vi "StringHeaderToCluster_v2(SubVI).vi"(8 "error in":errorcluster, 10 "UNDT_Cluster in":T1 {"Gain Coeff" format="%#_6e"; "Reserve 1" format="%02x"; "Mux TX" format="%02x"; "Mux RX" format="%02x"; "ScanDelay" format="%02x"; "PacketCounter" format="%08x"; "SamplingInterval" format="%#_6e"; "Lose Packet" format="%08x"; "EncodersParam2" format="%016x"; "EncodersParam1" format="%016x"; "CRC 8" format="%02x"; "N chanel" format="%02x"; "N tick" format="%02x"; "Ncycle" format="%04x"; "FrameFormatVersion" format="%02x"; "MagicWord" format="%.0x"}, 11 "string in":string) -> (0 "error out":errorcluster, 2 "UNDT_Cluster out":T1 {"Gain Coeff" format="%#_6e"; "Reserve 1" format="%02x"; "Mux TX" format="%02x"; "Mux RX" format="%02x"; "ScanDelay" format="%02x"; "PacketCounter" format="%08x"; "SamplingInterval" format="%#_6e"; "Lose Packet" format="%08x"; "EncodersParam2" format="%016x"; "EncodersParam1" format="%016x"; "CRC 8" format="%02x"; "N chanel" format="%02x"; "N tick" format="%02x"; "Ncycle" format="%04x"; "FrameFormatVersion" format="%02x"; "MagicWord" format="%.0x"})   [LabVIEW 2017]
uses:
  Control_EU/UNDT_ClusterPack (Type).ctl
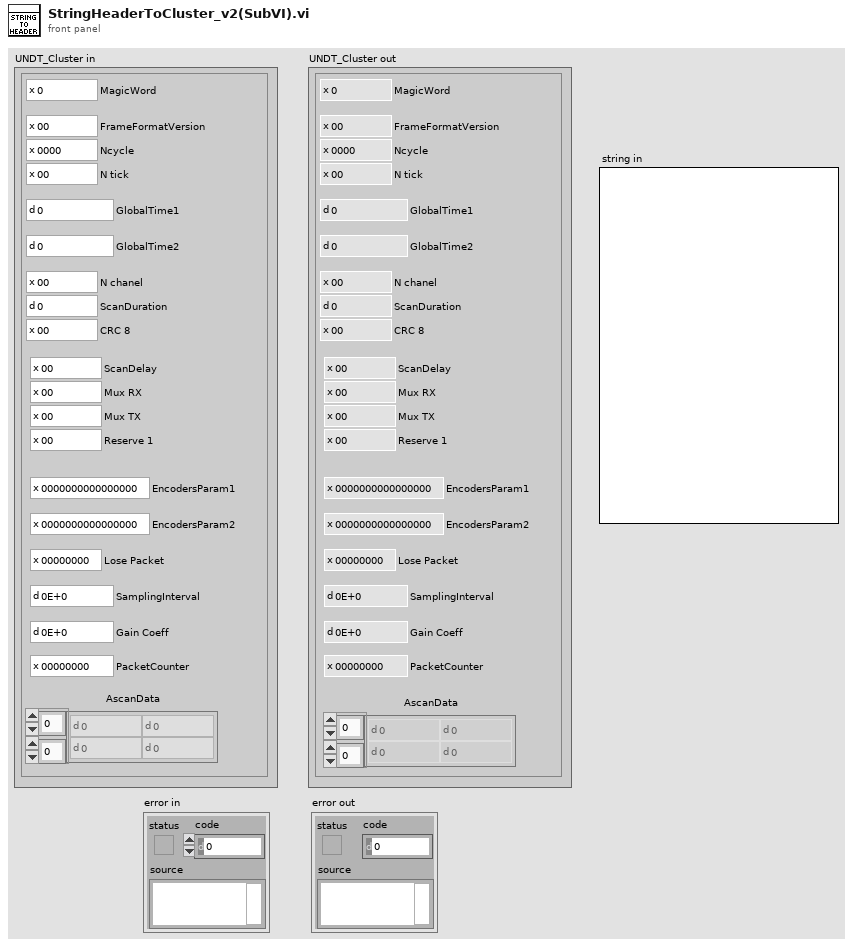
[diagram p1: front panel]
types:
  T1 = typedef "UNDT_ClusterPack (Type).ctl" = cluster{"MagicWord":u32, "FrameFormatVersion":u8, "Ncycle":u16, "N tick":u8, "GlobalTime1":u32, "GlobalTime2":u32, "N chanel":u8, "ScanDuration":u16, "CRC 8":u8, "EncodersParam1":u64, "EncodersParam2":u64, "Lose Packet":u32, "SamplingInterval":sgl, "PacketCounter":u32, "AscanData":dbl[][], "ScanDelay":u16, "Mux RX":u8, "Mux TX":u8, "Reserve 1":u8, "Gain Coeff":sgl}
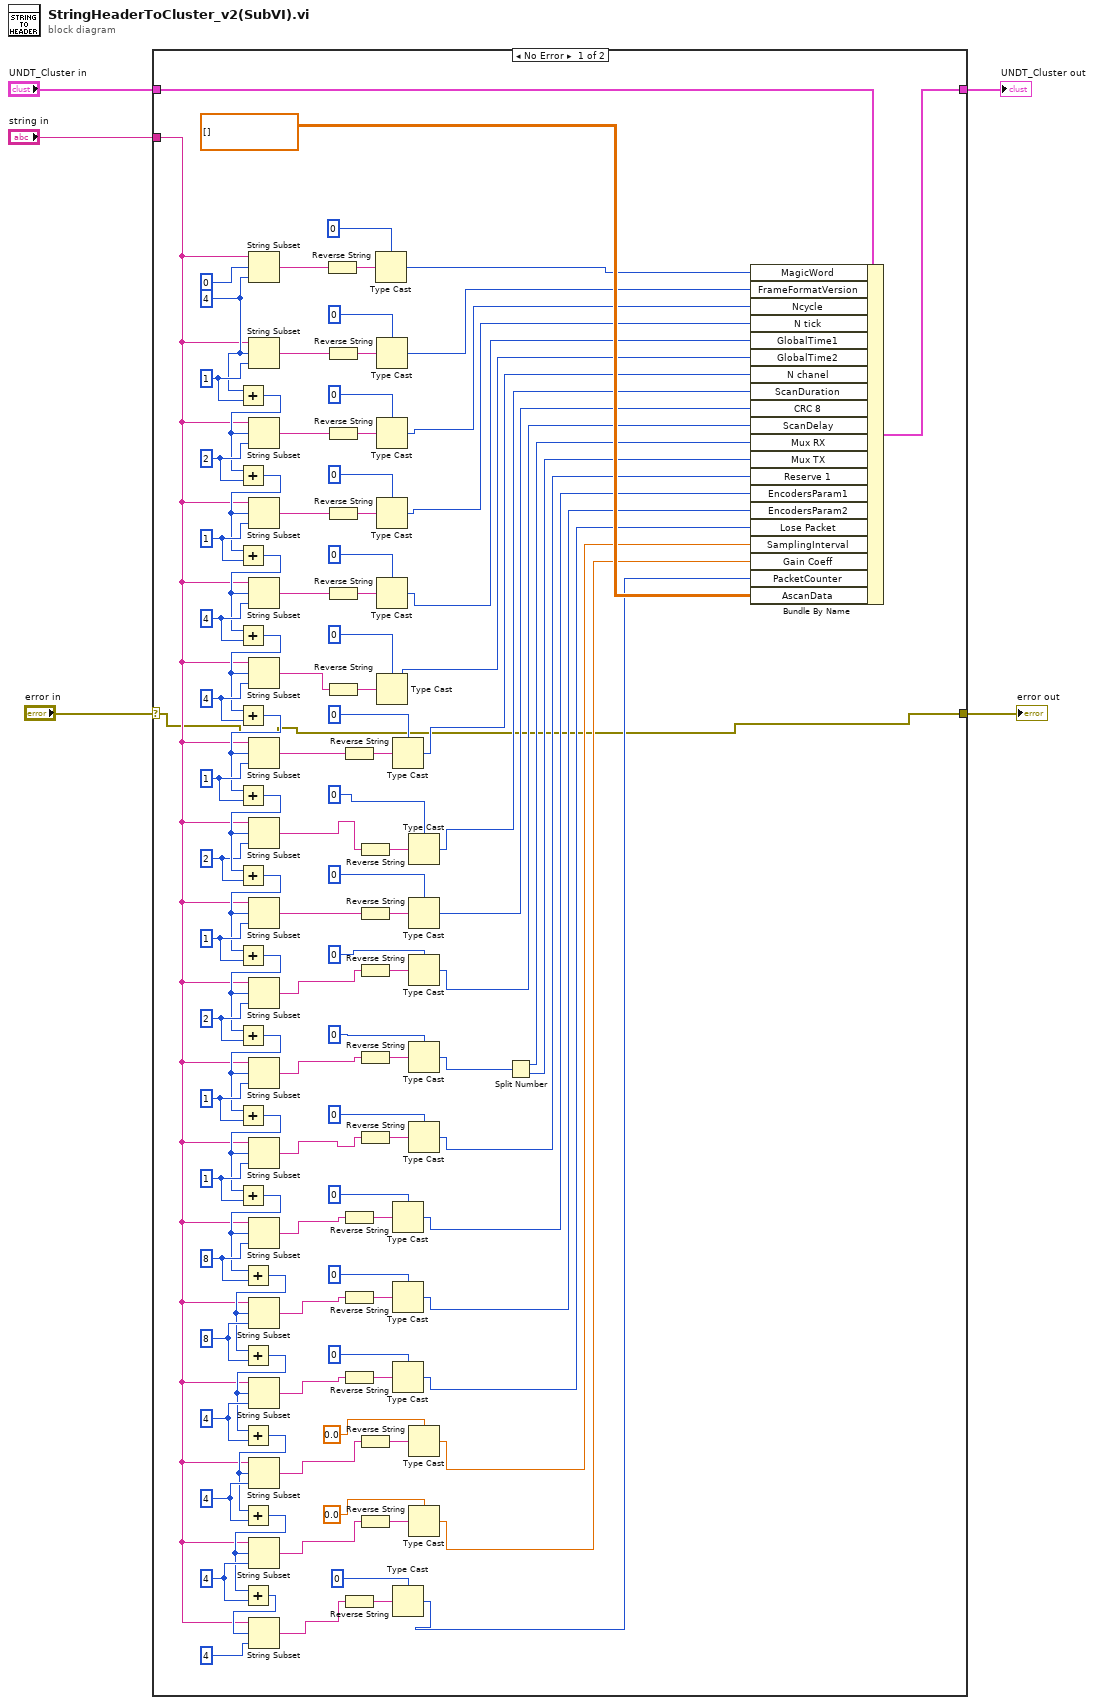
[diagram p0: block diagram]
diagram:
  n1 = case shown="No Error" "error in" {
    selector: "error in" -> [w6 w120]
    tunnel: "UNDT_Cluster in" -> [w86 w121]
    tunnel: [w85 w121] -> w4
    tunnel: "string in" -> [w79 _]
    tunnel: [w6 w120] -> w1
    frame No Error {
      w118 = 4 ("length (rest)")
      w116 = 4 ("length (rest)")
      w114 = 4 ("length (rest)")
      w112 = 8 ("length (rest)")
      w110 = 8 ("length (rest)")
      w109 = 1 ("length (rest)")
      w106 = 1 ("length (rest)")
      w104 = 2 ("length (rest)")
      w102 = 1 ("length (rest)")
      w99 = 2 ("length (rest)")
      w98 = 1 ("length (rest)")
      w96 = 4 ("length (rest)")
      w119 = 4 ("length (rest)")
      w94 = 1 ("length (rest)")
      w91 = 2 ("length (rest)")
      w89 = 1 ("length (rest)")
      w88 = 4 ("length (rest)")
      n2 = Add(x=w88, y=w89) -> (x+y=w90:i32)
      n3 = Add(x=w90, y=w91) -> (x+y=w92:i32)
      n4 = Add(x=w92, y=w94) -> (x+y=w93:i32)
      n5 = Add(x=w93, y=w119) -> (x+y=w95:i32)
      n6 = Add(x=w95, y=w96) -> (x+y=w97:i32)
      n7 = Add(x=w97, y=w98) -> (x+y=w100:i32)
      n8 = Add(x=w100, y=w99) -> (x+y=w101:i32)
      n9 = Add(x=w101, y=w102) -> (x+y=w103:i32)
      n10 = Add(x=w103, y=w104) -> (x+y=w105:i32)
      n11 = Add(x=w105, y=w106) -> (x+y=w107:i32)
      n12 = Add(x=w107, y=w109) -> (x+y=w108:i32)
      n13 = Add(x=w108, y=w110) -> (x+y=w111:i32)
      n14 = Add(x=w111, y=w112) -> (x+y=w113:i32)
      n15 = Add(x=w113, y=w114) -> (x+y=w115:i32)
      n16 = Add(x=w115, y=w116) -> (x+y=w117:i32)
      n17 = Add(x=w117, y=w118) -> (x+y=w81:i32)
      n18 = String Subset(string=w79, offset (0)=0, length (rest)=w88) -> (substring=w77:string)
      n19 = String Subset(string=w79, offset (0)=w88, length (rest)=w89) -> (substring=w69:string)
      n20 = String Subset(string=w79, offset (0)=w90, length (rest)=w91) -> (substring=w71:string)
      n21 = String Subset(string=w79, offset (0)=w92, length (rest)=w94) -> (substring=w63:string)
      n22 = String Subset(string=w79, offset (0)=w93, length (rest)=w119) -> (substring=w59:string)
      n23 = String Subset(string=w79, offset (0)=w95, length (rest)=w96) -> (substring=w55:string)
      n24 = String Subset(string=w79, offset (0)=w97, length (rest)=w98) -> (substring=w53:string)
      n25 = String Subset(string=w79, offset (0)=w100, length (rest)=w99) -> (substring=w48:string)
      n26 = String Subset(string=w79, offset (0)=w101, length (rest)=w102) -> (substring=w45:string)
      n27 = String Subset(string=w79, offset (0)=w103, length (rest)=w104) -> (substring=w41:string)
      n28 = String Subset(string=w79, offset (0)=w105, length (rest)=w106) -> (substring=w36:string)
      n29 = String Subset(string=w79, offset (0)=w107, length (rest)=w109) -> (substring=w33:string)
      n30 = String Subset(string=w79, offset (0)=w108, length (rest)=w110) -> (substring=w29:string)
      n31 = String Subset(string=w79, offset (0)=w111, length (rest)=w112) -> (substring=w25:string)
      n32 = String Subset(string=w79, offset (0)=w113, length (rest)=w114) -> (substring=w21:string)
      n33 = String Subset(string=w79, offset (0)=w115, length (rest)=w116) -> (substring=w17:string)
      n34 = String Subset(string=w79, offset (0)=w117, length (rest)=w118) -> (substring=w13:string)
      n35 = String Subset(string=w79, offset (0)=w81, length (rest)=4 ("length (rest)")) -> (substring=w9:string)
      n36 = Reverse String(1:w77) -> (0:w76:string)
      n37 = Reverse String(1:w69) -> (0:w74:string)
      n38 = Reverse String(1:w71) -> (0:w73:string)
      n39 = Reverse String(1:w63) -> (0:w66:string)
      n40 = Reverse String(1:w59) -> (0:w62:string)
      n41 = Reverse String(1:w55) -> (0:w58:string)
      n42 = Reverse String(1:w53) -> (0:w54:string)
      n43 = Reverse String(1:w29) -> (0:w30:string)
      n44 = Reverse String(1:w25) -> (0:w26:string)
      n45 = Reverse String(1:w21) -> (0:w22:string)
      n46 = Reverse String(1:w9) -> (0:w10:string)
      n47 = Reverse String(1:w48) -> (0:w50:string)
      n48 = Reverse String(1:w45) -> (0:w46:string)
      n49 = Reverse String(1:w41) -> (0:w42:string)
      n50 = Reverse String(1:w36) -> (0:w38:string)
      n51 = Reverse String(1:w33) -> (0:w34:string)
      n52 = Reverse String(1:w17) -> (0:w18:string)
      n53 = Reverse String(1:w13) -> (0:w14:string)
      n54 = Type Cast(type=u32 0 ("MagicWord 2"), x=w76) -> (*(type *) &x=w75:u32)
      n55 = Type Cast(type=u8 0 ("MagicWord 2"), x=w74) -> (*(type *) &x=w68:u8)
      n56 = Type Cast(type=u16 0 ("MagicWord 2"), x=w73) -> (*(type *) &x=w70:u16)
      n57 = Type Cast(type=u8 0 ("MagicWord 2"), x=w66) -> (*(type *) &x=w64:u8)
      n58 = Type Cast(type=u32 0 ("MagicWord 2"), x=w62) -> (*(type *) &x=w61:u32)
      n59 = Type Cast(type=u32 0 ("MagicWord 2"), x=w58) -> (*(type *) &x=w56:u32)
      n60 = Type Cast(type=u8 0 ("MagicWord 2"), x=w54) -> (*(type *) &x=w52:u8)
      n61 = Type Cast(type=u64 0 ("MagicWord 2"), x=w30) -> (*(type *) &x=w27:u64)
      n62 = Type Cast(type=u64 0 ("MagicWord 2"), x=w26) -> (*(type *) &x=w23:u64)
      n63 = Type Cast(type=u32 0 ("MagicWord 2"), x=w22) -> (*(type *) &x=w19:u32)
      n64 = Type Cast(type=u32 0 ("MagicWord 2"), x=w10) -> (*(type *) &x=w7:u32)
      n65 = Type Cast(type=u16 0 ("MagicWord 2"), x=w50) -> (*(type *) &x=w49:u16)
      n66 = Type Cast(type=u8 0 ("MagicWord 2"), x=w46) -> (*(type *) &x=w43:u8)
      n67 = Type Cast(type=u16 0 ("MagicWord 2"), x=w42) -> (*(type *) &x=w39:u16)
      n68 = Type Cast(type=u8 0 ("MagicWord 2"), x=w38) -> (*(type *) &x=w35:u8)
      n69 = Type Cast(type=u8 0 ("MagicWord 2"), x=w34) -> (*(type *) &x=w31:u8)
      n70 = Type Cast(type=sgl 0.0 ("MagicWord 2"), x=w18) -> (*(type *) &x=w15:sgl)
      n71 = Type Cast(type=sgl 0.0 ("MagicWord 2"), x=w14) -> (*(type *) &x=w11:sgl)
      n72 = Split Number(x=w35) -> (hi(x)=w83:u8, lo(x)=w82:u8)
      n73 = Bundle By Name(cluster=w86, "MagicWord"=w75, "FrameFormatVersion"=w68, "Ncycle"=w70, "N tick"=w64, "GlobalTime1"=w61, "GlobalTime2"=w56, "N chanel"=w52, "ScanDuration"=w49, "CRC 8"=w43, "ScanDelay"=w39, "Mux RX"=w83, "Mux TX"=w82, "Reserve 1"=w31, "EncodersParam1"=w27, "EncodersParam2"=w23, "Lose Packet"=w19, "SamplingInterval"=w15, "Gain Coeff"=w11, "PacketCounter"=w7, "AscanData"=dbl[][] [] ("Data1")) -> (w85:T1)
    }
    frame Error {
    }
  }
  "UNDT_Cluster out" <- w4
  "error out" <- w1
